vi "Write Exception list and Save all mode.vi"(8 "error in (no error)":errorcluster, 9 "Save all mode?":bool, 10 "Exception list":string[](array[string]), 11 "File Writer in":refnum<class "File Writer.lvclass">) -> (0 "error out":errorcluster, 3 "File Writer out":refnum<class "File Writer.lvclass">)   [LabVIEW 2020, in "File Writer.lvlib" / "File Writer.lvclass"]
doc: "Write exeption list and save all boolean to the class data."
uses:
  File Writer.lvclass
  File Writer.lvclass/File Writer.ctl
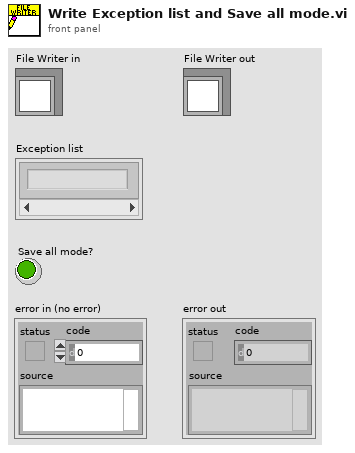
[diagram p1: front panel]
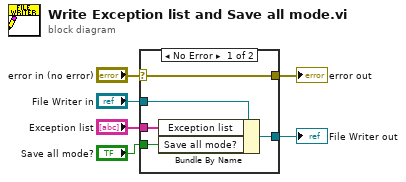
[diagram p0: block diagram]
diagram:
  n1 = case shown="No Error" "error in (no error)" {
    selector: "error in (no error)" -> [w11 w12]
    tunnel: [w11 w12] -> w5
    tunnel: [w9 w13] -> w3
    tunnel: "File Writer in" -> [w10 w13]
    tunnel: "Exception list" -> [w8 _]
    tunnel: "Save all mode?" -> [w7 _]
    frame No Error {
      n2 = Bundle By Name(cluster=w10, "Exception list"=w8, "Save all mode?"=w7) -> (w9:refnum<class "File Writer.lvclass">)
    }
    frame Error {
    }
  }
  "error out" <- w5
  "File Writer out" <- w3
